vi "P9.vi"() -> ()   [LabVIEW 2019]
panel:
  in  "Boolean":bool
  in  "stop":bool
  out "Slave 2":dbl(slide) scale=0.0..10.0
  out "Slave 1":dbl(slide) scale=0.0..10.0
  in  "Master Control":dbl(slide) scale=0.0..10.0
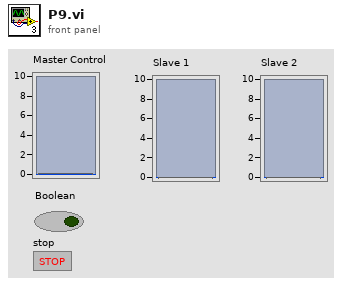
[diagram p1: front panel]
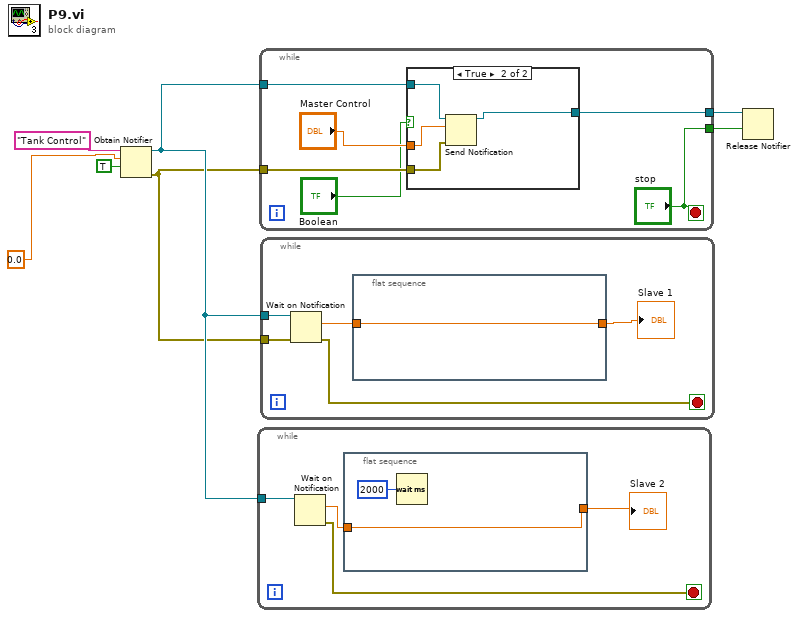
[diagram p0: block diagram]
diagram:
  n1 = Obtain Notifier(name (unnamed)="Tank Control", notification data type=0.0, create if not found? (T)=TRUE) -> (notifier out=w4:refnum<notifier>, error out=w1:errorcluster)  [unwired: 1 in, 1 out]
  n2 = while {
    tunnel: w4 -> [w11]
    stop <- w10 stop-if-true
    n3 = Wait on Notification(notifier=w11) -> (notification=w9:dbl, error out=w10:errorcluster)  [unwired: 3 in, 2 out]
    n4 = flat-sequence {
      tunnel: w9 -> [w12]
      tunnel: [w12] -> w8
      frame #0 {
        n5 = Wait (ms)(milliseconds to wait=u32 2000) -> ()  [unwired: 1 out]
      }
    }
    "Slave 2" <- w8
  }
  n6 = while {
    tunnel: w4 -> [w19]
    tunnel: [w17] -> w3
    tunnel: ["stop"] -> w2
    tunnel: w1 -> [w15]
    stop <- "stop" stop-if-true
    n7 = case shown="True" "Boolean" {
      tunnel: w19 -> [w20 w24]
      tunnel: "Master Control" -> [_ w23]
      tunnel: [w20 w22] -> w17
      tunnel: w15 -> [_ w21]
      frame False {
      }
      frame True {
        n8 = Send Notification(notification=w23, notifier=w24, error in (no error)=w21) -> (notifier out=w22:refnum<notifier>)  [unwired: 1 out]
      }
    }
  }
  n9 = while {
    tunnel: w4 -> [w29]
    tunnel: w1 -> [w28]
    stop <- w27 stop-if-true
    n10 = Wait on Notification(notifier=w29, error in (no error)=w28) -> (notification=w26:dbl, error out=w27:errorcluster)  [unwired: 2 in, 2 out]
    n11 = flat-sequence {
      tunnel: [w30] -> w25
      tunnel: w26 -> [w30]
      frame #0 {
      }
    }
    "Slave 1" <- w25
  }
  n12 = Release Notifier(notifier=w3, force destroy? (F)=w2) -> ()  [unwired: 1 in, 3 out]
